vi "Frame.GetSignalRefs.vi"(8 "error in (no error)":errorcluster, 11 "Frame Item Ref in":T1 format="%.0x") -> (0 "error out":errorcluster, 1 "Child Refs":T1[](array[typedef]) format="%.0x", 2 "Signal Collection Ref out":T1=18446744073709551615 format="%.0x", 3 "Original Frame Ref out":T1 format="%.0x")   [LabVIEW 2019, in "Diagnostics Addon System Explorer.lvlib"]
uses:
  Diagnostics Addon System Explorer.lvlib
  <vilib>/NI VeriStand/Custom Device API/Custom Device Item Ref.ctl
  Addon Shared/SubVIs/Constants.vi
  <vilib>/NI VeriStand/Custom Device Tools/Custom Device Utility Library/NI VeriStand - Search for Item by GUID.vi
  <vilib>/NI VeriStand/Custom Device API/Custom Device API.lvlib
  Addon Shared/Diagnostics Addon Shared.lvlib
  <vilib>/NI VeriStand/Custom Device Tools/Custom Device Utility Library/Custom Device Utility Library.lvlib
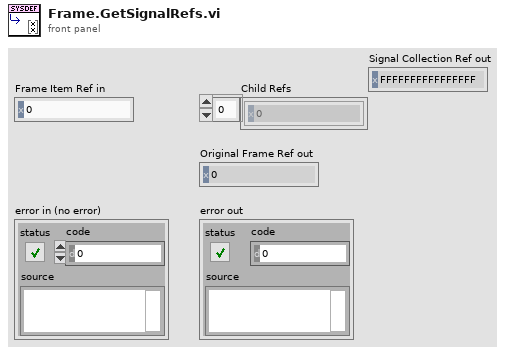
[diagram p1: front panel]
types:
  T1 = typedef "Custom Device API.lvlib/Custom Device Item Ref.ctl" = u64
  T2 = typedef "Custom Device API.lvlib/Custom Device Item Info.ctl" = cluster{"Name":string, "Is Channel":bool, "GUID":string, "Is Waveform":bool}
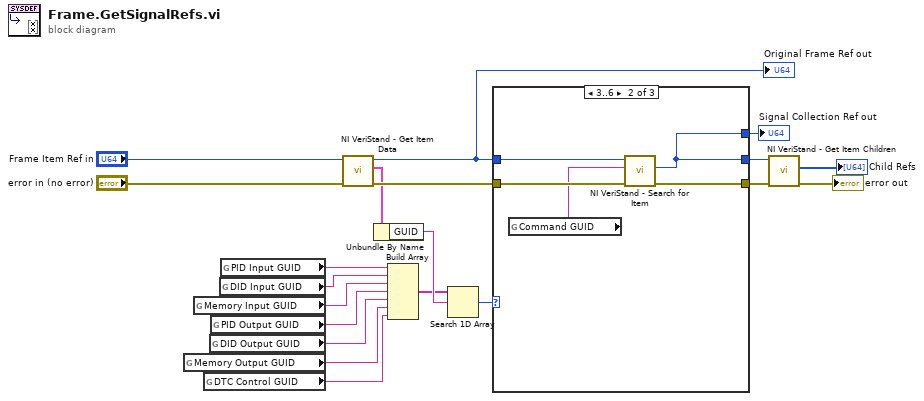
[diagram p0: block diagram]
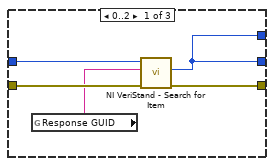
[diagram p2: hidden frame]
diagram:
  n1 = global read "Constants.vi" "Memory Output GUID"() -> (w13:string)
  n2 = global read "Constants.vi" "Memory Input GUID"() -> (w10:string)
  n3 = global read "Constants.vi" "DTC Control GUID"() -> (w1:string)
  n4 = global read "Constants.vi" "DID Output GUID"() -> (w12:string)
  n5 = global read "Constants.vi" "PID Output GUID"() -> (w11:string)
  n6 = global read "Constants.vi" "DID Input GUID"() -> (w9:string)
  n7 = global read "Constants.vi" "PID Input GUID"() -> (w8:string)
  n8 = call <vilib>:"NI VeriStand - Get Item Data.vi"("error in (no error)"="error in (no error)", "Item Ref in"="Frame Item Ref in") -> ("error out"=w17:errorcluster, "Item Info"=w5:T2, "Item Ref out"=w20:T1)  [unwired: 7 out]
  "Original Frame Ref out" <- w20
  n9 = Unbundle By Name(w5) -> ("GUID"=w15:string)
  n10 = Build Array(w8, w9, w10, w11, w12, w13, w1) -> (w14:string[])
  n11 = Search 1D Array(1D array=w14, element=w15) -> (index of element=w16:i32)  [unwired: 1 in]
  n12 = case shown="3..6" w16 {
    tunnel: w17 -> [w25 w30 w32]
    tunnel: w20 -> [w24 w29 w31]
    tunnel: [w22 w28 w32] -> w18
    tunnel: [w21 w26 w31] -> w19
    tunnel: [w21 w26 w31] -> w2
    frame 0..2 {
      n13 = global read "Constants.vi" "Response GUID"() -> (w23:string)
      n14 = call-poly <vilib>:"NI VeriStand - Search for Item.vi"("error in"=w25, "Item GUID"=w23, "Section Ref in"=w24) -> ("error out"=w22:errorcluster, "Item Ref"=w21:T1)  [unwired: 5 in, 2 out]
    }
    frame 3..6 {
      n15 = global read "Constants.vi" "Command GUID"() -> (w27:string)
      n16 = call-poly <vilib>:"NI VeriStand - Search for Item.vi"("error in"=w30, "Item GUID"=w27, "Section Ref in"=w29) -> ("error out"=w28:errorcluster, "Item Ref"=w26:T1)  [unwired: 5 in, 2 out]
    }
    frame Default {
    }
  }
  "Signal Collection Ref out" <- w2
  n17 = call <vilib>:"NI VeriStand - Get Item Children.vi"("error in (no error)"=w18, "Item Ref in"=w19) -> ("error out"=→"error out":errorcluster, "Child Refs"=→"Child Refs":T1[])  [unwired: 6 in, 2 out]
